vi "Failure Message With Application.vi"() -> ()   [LabVIEW 2017, in "Assertion.Tests.lvlib" / "Assert Not Refnum.lvlib"]
uses:
  Assert Not Refnum.lvlib
  Assertion/Assertion.lvlib
panel:
  out "error out":errorcluster
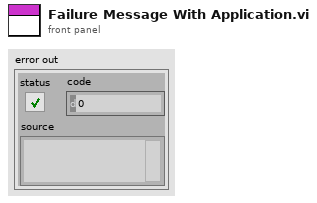
[diagram p1: front panel]
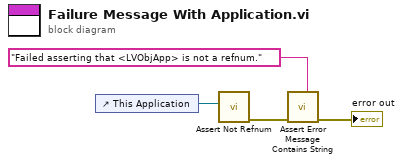
[diagram p0: block diagram]
diagram:
  n1 = control-ref of="This Application"() -> (w1:refnum<vi>)
  n2 = call "Assert Not Refnum.vi"("Refnum"=w1) -> ("error out"=w4:errorcluster)  [unwired: 10 in]
  n3 = call "Assert Error Message Contains String.vi"("Expected"="Failed asserting that <LVObjApp> is not a refnum.", "error in (no error)"=w4) -> ("error out"=→"error out":errorcluster)  [unwired: 9 in]
